vi "Get Duration of Current State.vi"(10 "samples generated at state":u64, 11 "signal configuration":refnum<class "SV Signal.lvclass">) -> (2 "current state duration [s]":dbl, 3 "signal configuration":refnum<class "SV Signal.lvclass">)   [LabVIEW 2017, in "SV Signal.lvclass"]
uses:
  <vilib>/addons/_NISVFA/_Generation/Signal Generation/SV Signal/SV Signal.lvclass
  <vilib>/addons/_NISVFA/_Generation/Signal Generation/SV Signal/SV Signal.lvclass/SV Signal.ctl
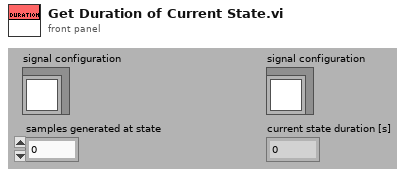
[diagram p1: front panel]
types:
  T1 = typedef "SV Signal.lvclass/sv_Generation State.ctl" = enum16{"Idle", "Ramp Up", "Pre-Measurement Settling", "Measurement", "Post-Measurement Settling", "Discrete Sweep Transition", "Ramp Down", "Update"}
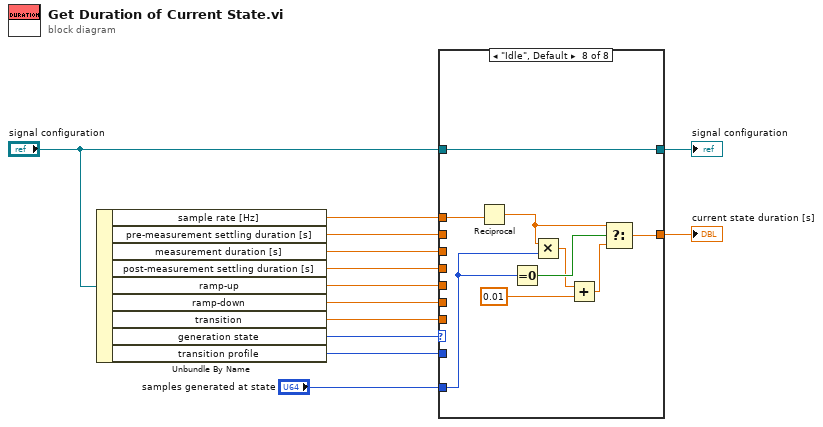
[diagram p0: block diagram]
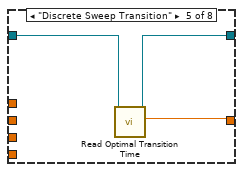
[diagram p7: hidden frame]
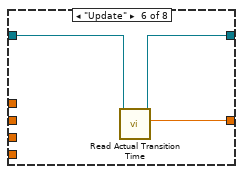
[diagram p8: hidden frame]
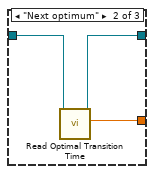
[diagram p10: hidden frame]
diagram:
  n1 = Unbundle By Name("signal configuration") -> ("sample rate [Hz]"=w2:dbl, "pre-measurement settling duration [s]"=w8:dbl, "measurement duration [s]"=w7:dbl, "post-measurement settling duration [s]"=w6:dbl, "ramp-up"=w10:dbl, "ramp-down"=w11:dbl, "transition"=w12:dbl, "generation state"=w13:T1, "transition profile"=w3:enum16{"Immediate", "Next optimum", "Ramp"})
  n2 = case shown="\"Idle\", Default" w13 {
    tunnel: w10 -> [w16 _ _ _ _ _ _ _]
    tunnel: w8 -> [_ w20 _ _ _ _ _ _]
    tunnel: w7 -> [_ _ w22 _ _ _ _ _]
    tunnel: w6 -> [_ _ _ w24 _ _ _ _]
    tunnel: w11 -> [_ _ _ _ _ _ w33 _]
    tunnel: [w15 w20 w22 w24 w25 w29 w34 w49] -> w9
    tunnel: w12 -> [_ _ _ _ _ _ _ _]
    tunnel: "signal configuration" -> [w17 w19 w21 w23 w27 w30 w32 w50]
    tunnel: [w17 w19 w21 w23 w26 w28 w31 w50] -> w4
    tunnel: w3 -> [w14 _ _ _ _ _ w35 _]
    tunnel: "samples generated at state" -> [_ _ _ _ _ _ _ w46]
    tunnel: w2 -> [_ _ _ _ _ _ _ w48]
    frame "Ramp Up" {
      n3 = case shown="\"Ramp\"" w14 {
        tunnel: [_ w18] -> w15
        tunnel: w16 -> [_ w18]
        frame "Immediate", Default {
        }
        frame "Ramp" {
        }
      }
    }
    frame "Pre-Measurement Settling" {
    }
    frame "Measurement" {
    }
    frame "Post-Measurement Settling" {
    }
    frame "Discrete Sweep Transition" {
      n4 = call <vilib>:"Read Optimal Transition Time.vi"("signal configuration in"=w27) -> ("optimal transition time"=w25:dbl, "signal configuration out"=w26:refnum<class "SV Signal.lvclass">)  [unwired: 8 in, 1 out]
    }
    frame "Update" {
      n5 = call <vilib>:"Read Actual Transition Time.vi"("signal configuration in"=w30) -> ("actual transition time"=w29:dbl, "signal configuration out"=w28:refnum<class "SV Signal.lvclass">)  [unwired: 8 in, 1 out]
    }
    frame "Ramp Down" {
      n6 = case shown="\"Immediate\", Default" w35 {
        tunnel: [_ w37 w41] -> w34
        tunnel: w33 -> [_ _ w41]
        tunnel: w32 -> [w36 w39 w40]
        tunnel: [w36 w38 w40] -> w31
        frame "Immediate", Default {
        }
        frame "Next optimum" {
          n7 = call <vilib>:"Read Optimal Transition Time.vi"("signal configuration in"=w39) -> ("optimal transition time"=w37:dbl, "signal configuration out"=w38:refnum<class "SV Signal.lvclass">)  [unwired: 8 in, 1 out]
        }
        frame "Ramp" {
        }
      }
    }
    frame "Idle", Default {
      n8 = Reciprocal(x=w48) -> (1/x=w42:dbl)
      n9 = Equal To 0?(x=w46) -> (x = 0?=w47:bool)
      n10 = Multiply(x=w42, y=w46) -> (x*y=w44:dbl)
      n11 = Add(x=w44, y=0.01 ("x")) -> (x+y=w43:dbl)
      n12 = Select(t=w42, s=w47, f=w43) -> (s? t:f=w49:dbl)
    }
  }
  "current state duration [s]" <- w9
  "signal configuration" <- w4
